vi "arduinoSerialComm.vi"() -> ()   [LabVIEW 2019]
uses:
  <vilib>/Utility/miscctls.llb/LVComboBoxStrsAndValuesArrayTypeDef.ctl
  <vilib>/Instr/_visa.llb/VISA Configure Serial Port (Instr).vi
panel:
  in  "Command":string(combo)
  in  "Error In":errorcluster
  in  "millisecond timer value":u32=1000
  out "Recieve Log":string
  out "Serial Settings:Number of Bytes at Serial Port":u32
  in  "Turn On":bool
  in  "Stop Button":bool
  in  "Baud Rate":u32=9600
  in  "COM Port":refnum<visa-resource-name>="COM4"
  out "Available?":bool
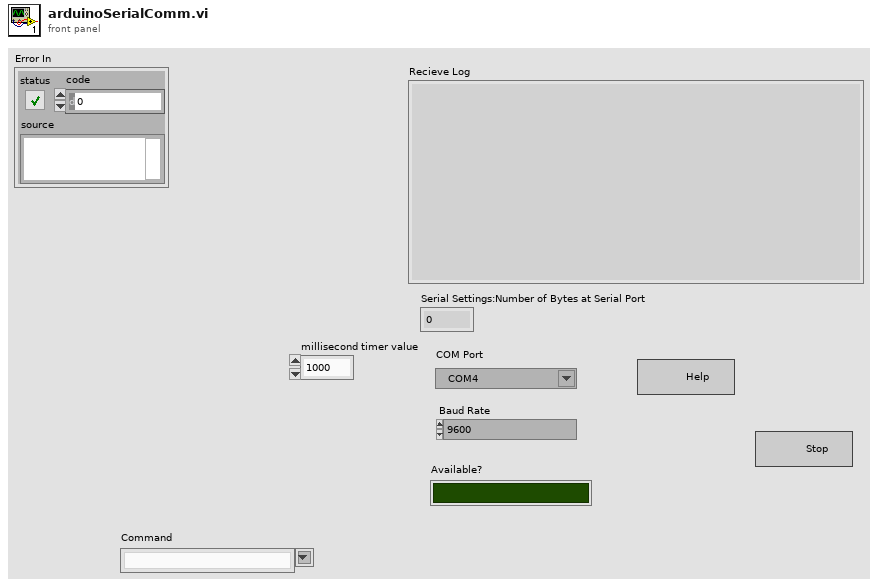
[diagram p1: front panel]
types:
  T1 = typedef "LVComboBoxStrsAndValuesArrayTypeDef.ctl" = cluster{"String":string, "Value":string}[]
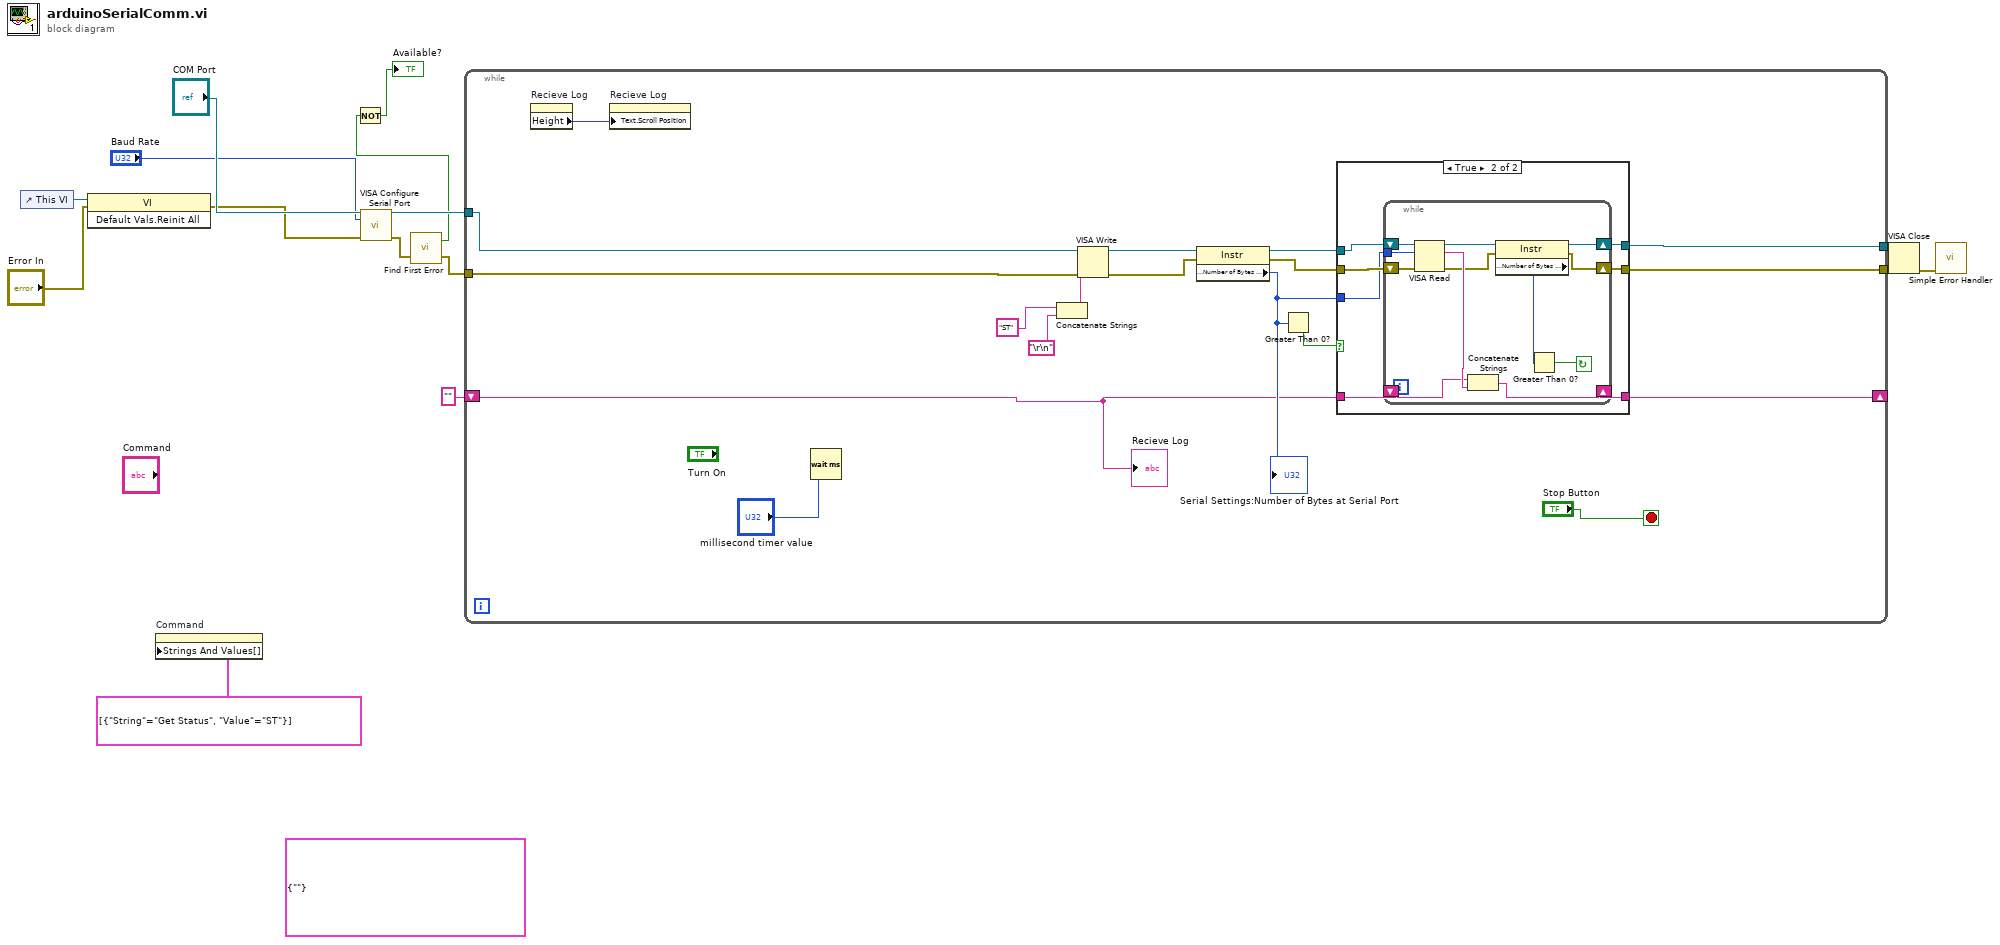
[diagram p0: block diagram]
diagram:
  (unwired) cluster{string} {""}
  n1 = control-ref of="This VI"() -> (w12:refnum<vi>)
  n2 = invoke class="VI" method="Default Vals.Reinit All"(reference=w12, error in="Error In") -> (error out=w8:errorcluster)  [unwired: 1 in, 2 out]
  n3 = property on="Command" class="CmbBox"("Strings And Values[]"=T1 [{"String"="Get Status", "Value"="ST"}] ("Strings And Values []")) -> ()  [unwired: 2 in, 2 out]
  n4 = call-poly "VISA Configure Serial Port"("VISA resource name"="COM Port", "baud rate (9600)"="Baud Rate", "error in (no error)"=w8) -> ("VISA resource name out"=w7:refnum<visa-resource-name>, "error out"=w6:errorcluster)  [unwired: 11 in]
  n5 = call <vilib>:"Find First Error.vi"("error in (no error)"=w6) -> ("error out"=w5:errorcluster, "error?"=w4:bool)  [unwired: 3 in]
  n6 = Not(x=w4) -> (.not. x?=→"Available?":bool)
  n7 = while {
    tunnel: [w28] -> w14
    tunnel: [w27] -> w15
    shift-right: [w23] -> _
    shift-left: "" -> [w19]
    tunnel: w7 -> [w21]
    tunnel: w5 -> [w20]
    stop <- "Stop Button" stop-if-true
    n8 = property on="Recieve Log" class="Str"() -> ("Height"=w22:u32)  [unwired: 2 in, 2 out]
    n9 = property on="Recieve Log" class="Str"("Text.Scroll Position"=w22) -> ()  [unwired: 2 in, 2 out]
    n10 = Wait (ms)(milliseconds to wait="millisecond timer value") -> ()  [unwired: 1 out]
    n11 = Concatenate Strings("ST" ("write buffer"), "\r\n") -> (w18:string)
    n12 = VISA Write(VISA resource name=w21, write buffer=w18, error in (no error)=w20) -> (VISA resource name out=w33:refnum<visa-resource-name>, error out=w32:errorcluster)  [unwired: 1 out]
    n13 = property class="Instr"(reference=w33, error in=w32) -> (reference out=w29:refnum<visa-resource-name>, error out=w30:errorcluster, "Serial Settings:Number of Bytes at Serial Port"=w26:u32)
    "Serial Settings:Number of Bytes at Serial Port" <- w26
    n14 = Greater Than 0?(x=w26) -> (x > 0?=w31:bool)
    n15 = case shown="True" w31 {
      tunnel: w29 -> [w36 w43]
      tunnel: w30 -> [w35 w41]
      tunnel: [w36 w42] -> w28
      tunnel: [w35 w40] -> w27
      tunnel: w26 -> [_ w39]
      tunnel: w19 -> [w34 w38]
      tunnel: [w34 w37] -> w23
      frame False {
      }
      frame True {
        n16 = while {
          tunnel: w39 -> [w53]
          shift-right: [w44] -> w42
          shift-left: w43 -> [w55]
          shift-right: [w48] -> w40
          shift-left: w41 -> [w54]
          shift-right: [w50] -> w37
          shift-left: w38 -> [w51]
          stop <- w47 continue-if-true
          n17 = VISA Read(VISA resource name=w55, byte count=w53, error in (no error)=w54) -> (VISA resource name out=w45:refnum<visa-resource-name>, read buffer=w52:string, error out=w49:errorcluster)  [unwired: 1 out]
          n18 = Concatenate Strings(w51, w52) -> (w50:string)
          n19 = property class="Instr"(reference=w45, error in=w49) -> (reference out=w44:refnum<visa-resource-name>, error out=w48:errorcluster, "Serial Settings:Number of Bytes at Serial Port"=w46:u32)
          n20 = Greater Than 0?(x=w46) -> (x > 0?=w47:bool)
        }
      }
    }
    "Recieve Log" <- w19
  }
  n21 = VISA Close(VISA resource name=w14, error in (no error)=w15) -> (error out=w13:errorcluster)
  n22 = call <vilib>:"Simple Error Handler.vi"("error in (no error)"=w13) -> ()  [unwired: 4 in, 5 out]
